vi "Make Bar Plots - Adv. Plotting.vi"(0 "Picture in":refnum<vi>, 1 "Save Plot?":bool, 2 "Save Path":path=path "", 5 "Labels":string[](array[string]), 7 "Legend Title":string="SPARC", 9 "SPARC":dbl[](array[numeric]), 11 "error in (no error)":errorcluster, 12 "Title":string, 13 "Y Min":dbl=-7.0 format="%#_13g") -> (4 "Picture":picture, 15 "error out":errorcluster)   [LabVIEW 2020]
uses:
  <vilib>/Heliosphere Research LLC/Advanced Plotting Toolkit/api_figure/TicksProperties.ctl
  <vilib>/Heliosphere Research LLC/Advanced Plotting Toolkit/properties/Text.ctl
  <vilib>/Heliosphere Research LLC/Advanced Plotting Toolkit/typedefs/PlotColor.ctl
  <vilib>/Heliosphere Research LLC/Advanced Plotting Toolkit/properties/Text_FontSize.ctl
  <vilib>/Heliosphere Research LLC/Advanced Plotting Toolkit/properties/Text_FontStyle.ctl
  <vilib>/Heliosphere Research LLC/Advanced Plotting Toolkit/api_core/NewPlotProperties.ctl
  <vilib>/Heliosphere Research LLC/Advanced Plotting Toolkit/api_annotations/LabelProperties.ctl
  <vilib>/Heliosphere Research LLC/Advanced Plotting Toolkit/Advanced Plotting Toolkit.lvlib
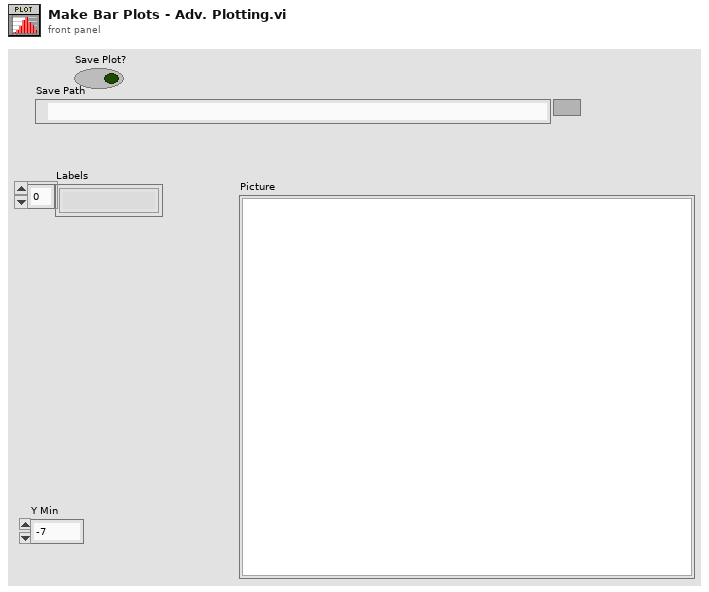
[diagram p1: front panel]
types:
  T1 = typedef "Advanced Plotting Toolkit.lvlib/LabelProperties.ctl" = cluster{"Text":T2}
  T2 = typedef "Advanced Plotting Toolkit.lvlib/Text.ctl" = cluster{"Color":T3, "Background Color":T3, "Font Size (points)":T4, "Font Style":T5, "Rotation Angle":dbl}
  T3 = typedef "Advanced Plotting Toolkit.lvlib/PlotColor.ctl" = u32
  T4 = typedef "Advanced Plotting Toolkit.lvlib/Text_FontSize.ctl" = i32
  T5 = typedef "Advanced Plotting Toolkit.lvlib/Text_FontStyle.ctl" = enum16{"Automatic", "Normal", "Italic", "Bold"}
  T6 = typedef "Advanced Plotting Toolkit.lvlib/NewPlotProperties.ctl" = cluster{"Background Color":T3, "Axis Background":T3, "Left Margin":dbl, "Right Margin":dbl, "Bottom Margin":dbl, "Top Margin":dbl, "Aspect Ratio":dbl}
  T7 = typedef "Advanced Plotting Toolkit.lvlib/TicksProperties.ctl" = cluster{"Text":T2}
  T8 = typedef "Advanced Plotting Toolkit.lvlib/PlotID.ctl" = i32
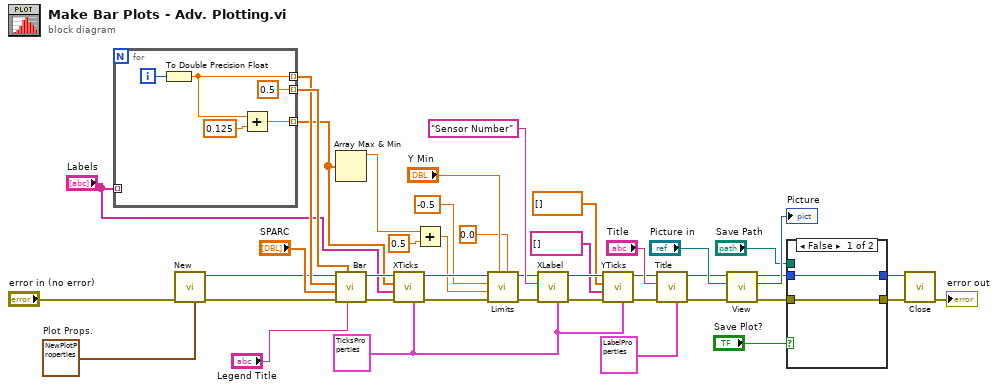
[diagram p0: block diagram]
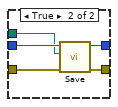
[diagram p2: hidden frame]
diagram:
  w35 = T6 {"Background Color"=2147483647, "Axis Background"=2147483647, "Left Margin"=nan, "Right Margin"=nan, "Bottom Margin"=0.125, "Top Margin"=nan, "Aspect Ratio"=nan}  # Plot Props.
  w3 = T7 {"Text"={"Color"=0, "Background Color"=16777215, "Font Size (points)"=-3, "Font Style"=enum."Bold", "Rotation Angle"=0.0}} ("X Ticks")
  n1 = for {
    tunnel: [w45] -> w40 mode=indexing
    tunnel: [w46] -> w26 mode=indexing
    tunnel: [0.5 ("Numeric")] -> w41 mode=indexing
    tunnel: "Labels" -> [_] mode=indexing
    i -> [w48]
    n2 = To Double Precision Float(number=w48) -> (double precision float=w45:dbl)
    n3 = Add(x=w45, y=0.125) -> (x+y=w46:dbl)
  }
  n4 = call <vilib>:"New.vi"("Properties"=w35, "error in (no error)"="error in (no error)") -> ("error out"=w34:errorcluster, "Plot ID"=w32:T8)  [unwired: 8 in]
  n5 = Array Max & Min(array=w26) -> (max value=w25:dbl)  [unwired: 3 out]
  n6 = call <vilib>:"Bar.vi"("Legend Title"="Legend Title", "Bar Widths"=w41, "error in (no error)"=w34, "Bar Lengths"="SPARC", "X Coordinates"=w40, "Plot ID"=w32) -> ("error out"=w39:errorcluster, "Plot ID Out"=w38:T8)  [unwired: 4 in]
  n7 = call <vilib>:"XTicks.vi"("Properties"=w3, "error in (no error)"=w39, "Tick Labels"="Labels", "Tick Locations"=w26, "Plot ID"=w38) -> ("error out"=w28:errorcluster, "Plot ID Out"=w29:T8)  [unwired: 5 in]
  n8 = Add(x=w25, y=0.5) -> (x+y=w24:dbl)
  n9 = call <vilib>:"Limits.vi"("Y Max"=0.0, "Y Min"="Y Min", "error in (no error)"=w28, "X Max"=w24, "X Min"=-0.5, "Plot ID"=w29) -> ("error out"=w21:errorcluster, "Plot ID Out"=w22:T8)  [unwired: 4 in]
  n10 = call <vilib>:"XLabel.vi"("Properties"=w3, "error in (no error)"=w21, "Label"="Sensor Number", "Plot ID"=w22) -> ("error out"=w18:errorcluster, "Plot ID out"=w19:T8)  [unwired: 6 in]
  n11 = call <vilib>:"YTicks.vi"("Properties"=w3, "error in (no error)"=w18, "Tick Labels"=string[] [], "Tick Locations"=dbl[] [], "Plot ID"=w19) -> ("error out"=w14:errorcluster, "Plot ID Out"=w15:T8)  [unwired: 5 in]
  n12 = call <vilib>:"Title.vi"("Properties"=T1 {"Text"={"Color"=2147483647, "Background Color"=2147483647, "Font Size (points)"=-4, "Font Style"=enum."Bold", "Rotation Angle"=nan}}, "error in (no error)"=w14, "Title"="Title", "Plot ID"=w15) -> ("error out"=w4:errorcluster, "Plot ID out"=w5:T8)  [unwired: 6 in]
  n13 = call <vilib>:"View.vi"("error in (no error)"=w4, "Ref for Sizing"="Picture in", "Plot ID"=w5) -> ("error out"=w10:errorcluster, "Picture"=→"Picture":picture, "Plot ID Out"=w11:T8)  [unwired: 6 in]
  n14 = case shown="False" "Save Plot?" {
    tunnel: w11 -> [w49 w55]
    tunnel: w10 -> [w50 w54]
    tunnel: [w49 w53] -> w9
    tunnel: [w50 w52] -> w8
    tunnel: "Save Path" -> [_ w51]
    frame False {
    }
    frame True {
      n15 = call <vilib>:"Save.vi"("error in (no error)"=w54, "Path"=w51, "Plot ID In"=w55) -> ("error out"=w52:errorcluster, "Plot ID Out"=w53:T8)  [unwired: 7 in]
    }
  }
  n16 = call <vilib>:"Close.vi"("error in (no error)"=w8, "Plot ID"=w9) -> ("error out"=→"error out":errorcluster)  [unwired: 9 in]
